vi "ShooterRollingAverageDistance.vi"(11 "Distance (ft)":dbl) -> (3 "distanceMean":dbl)   [LabVIEW 2015]
uses:
  <vilib>/Analysis/baseanly.llb/Mean (DBL).vi
  <vilib>/Analysis/NI_AALBase.lvlib
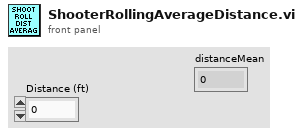
[diagram p1: front panel]
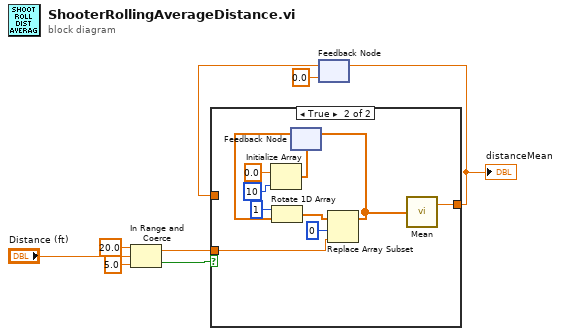
[diagram p0: block diagram]
diagram:
  n1 = In Range and Coerce(upper limit=20.0, x="Distance (ft)", lower limit=5.0) -> (coerced(x)=w5:dbl, In Range?=w2:bool)
  n2 = feedback #1(0.0 ("mean")) -> (w7:dbl)
  n3 = case shown="True" w2 {
    tunnel: w5 -> [_ w12]
    tunnel: [w9 w10] -> w6
    tunnel: w7 -> [w9 _]
    frame False {
    }
    frame True {
      n4 = Initialize Array(0.0 ("element"), 10 ("dimension size")) -> (w13:dbl[])
      n5 = feedback #2(w13) -> (w14:dbl[])
      n6 = Rotate 1D Array(1:w14, 2:1 ("n")) -> (0:w16:dbl[])
      n7 = Replace Array Subset(array=w16, new element=w12, index=0) -> (w11:dbl[])
      n8 = feedback-in #2(w11) -> ()
      n9 = call-poly <vilib>:"Mean.vi"("X"=w11) -> ("mean"=w10:dbl)  [unwired: 1 out]
    }
  }
  "distanceMean" <- w6
  n10 = feedback-in #1(w6) -> ()
